vi "Affichage - 2 cam - 1P - 2.vi"(7 "Image 2D 2":picture, 8 "Couleur rectangle":u32(colorbox)=16775680, 9 "Caméra D":T1, 10 "Choix cam":u16, 11 "Caméra G":T1) -> (2 "Image 2D":picture)   [LabVIEW 2013]
panel:
  # "Affichage"
  # "Pour un rectangle"
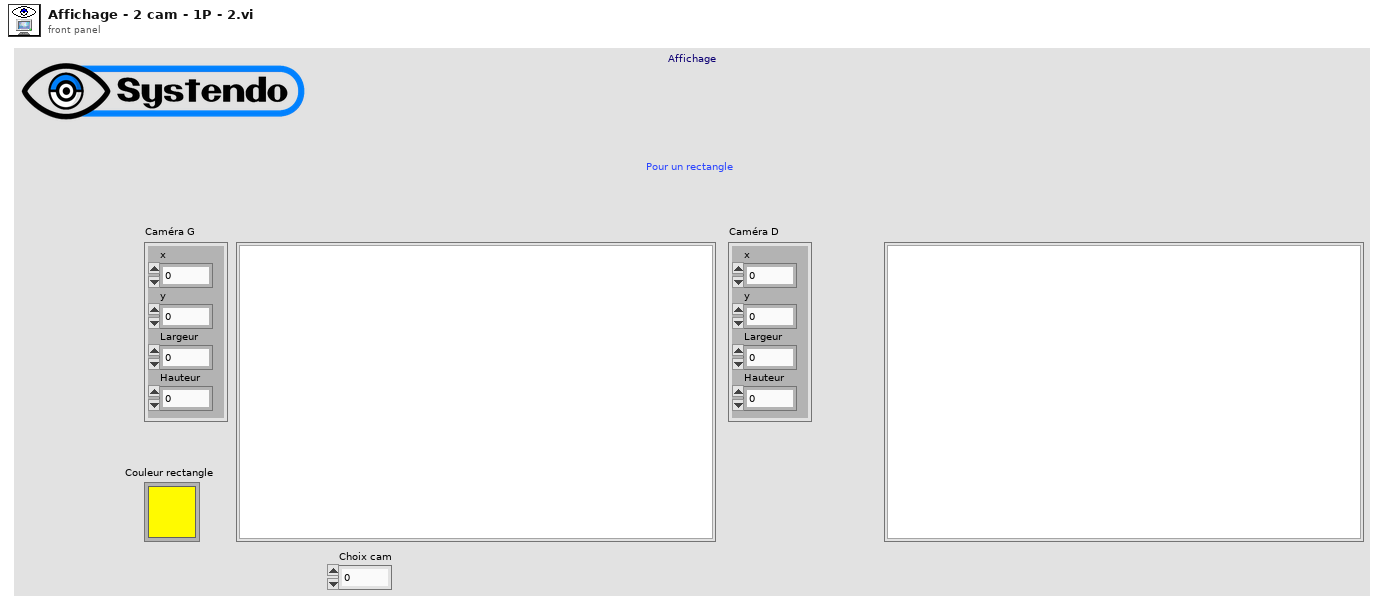
[diagram p1: front panel]
types:
  T1 = cluster{"x":i16, "y":i16, "Largeur":i16, "Hauteur":i16}
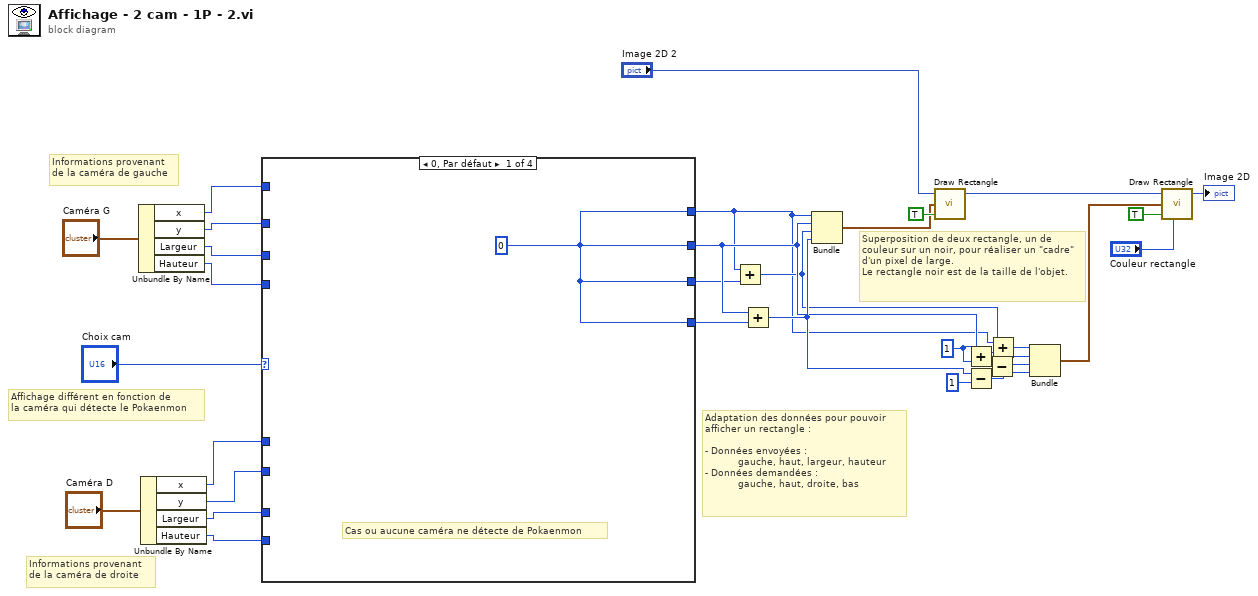
[diagram p0: block diagram]
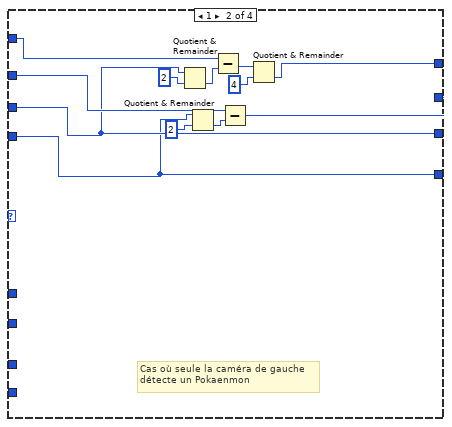
[diagram p2: hidden frame]
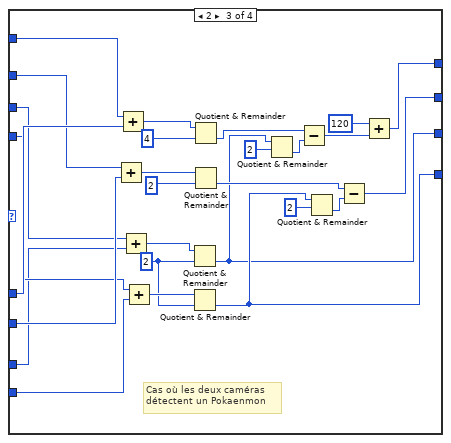
[diagram p3: hidden frame]
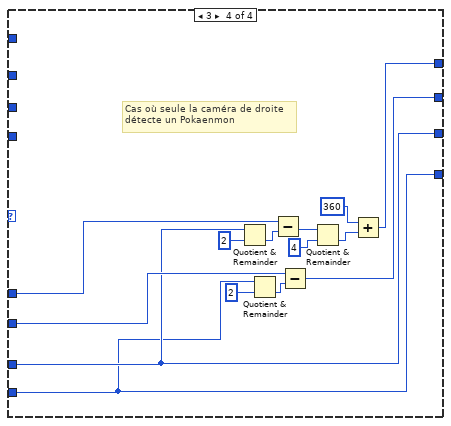
[diagram p4: hidden frame]
diagram:
  w10 = i16 1 ("y")
  w7 = i16 1 ("y")
  # "Superposition de deux rectangle, un de couleur sur un noir, pour réaliser un \"cadre\" d'un pixel de large.\nLe rectangle noir est de la taille de l'objet."
  # "Adaptation des données pour pouvoir\nafficher un rectangle :\n\n- Données envoyées :\n           gauche, haut, largeur, hauteur\n- Données demandées :\n           gauche, haut, droite, bas"
  # "Informations provenant\nde la caméra de droite"
  # "Informations provenant\nde la caméra de gauche"
  # "Affichage différent en fonction de\nla caméra qui détecte le Pokaenmon"
  n1 = Unbundle By Name("Caméra G") -> ("x"=w23:i16, "y"=w22:i16, "Largeur"=w21:i16, "Hauteur"=w20:i16)
  n2 = Unbundle By Name("Caméra D") -> ("x"=w16:i16, "y"=w17:i16, "Largeur"=w18:i16, "Hauteur"=w19:i16)
  n3 = case shown="0, Par défaut" "Choix cam" {
    tunnel: [w32 w36 w54 w81] -> w27
    tunnel: [w32 w42 w53 w83] -> w30
    tunnel: [w32 w40 w45 w76] -> w26
    tunnel: [w32 w34 w51 w73] -> w29
    tunnel: w16 -> [_ _ w64 w84]
    tunnel: w17 -> [_ _ w62 w85]
    tunnel: w18 -> [_ _ w59 w76]
    tunnel: w19 -> [_ _ w61 w73]
    tunnel: w20 -> [_ w34 w60 _]
    tunnel: w21 -> [_ w40 w58 _]
    tunnel: w22 -> [_ w43 w63 _]
    tunnel: w23 -> [_ w44 w65 _]
    frame 0, Default {
      w32 = 0
      # "Cas ou aucune caméra ne détecte de Pokaenmon"
    }
    frame 1 {
      # "Cas où seule la caméra de gauche\ndétecte un Pokaenmon"
      n4 = Quotient & Remainder(x=w40, y=u16 2) -> (floor(x/y)=w39:u16)  [unwired: 1 out]
      n5 = Quotient & Remainder(x=w34, y=u16 2) -> (floor(x/y)=w33:u16)  [unwired: 1 out]
      n6 = Subtract(x=w44, y=w39) -> (x-y=w37:u16)
      n7 = Subtract(x=w43, y=w33) -> (x-y=w42:u16)
      n8 = Quotient & Remainder(x=w37, y=u16 4) -> (floor(x/y)=w36:u16)  [unwired: 1 out]
    }
    frame 2 {
      w66 = i16 2 ("y")
      # "Cas où les deux caméras\ndétectent un Pokaenmon"
      n9 = Add(x=w63, y=w62) -> (x+y=w70:i16)
      n10 = Add(x=w65, y=w64) -> (x+y=w71:i16)
      n11 = Add(x=w58, y=w59) -> (x+y=w68:i16)
      n12 = Add(x=w60, y=w61) -> (x+y=w67:i16)
      n13 = Quotient & Remainder(x=w68, y=w66) -> (floor(x/y)=w45:i16)  [unwired: 1 out]
      n14 = Quotient & Remainder(x=w67, y=w66) -> (floor(x/y)=w51:i16)  [unwired: 1 out]
      n15 = Quotient & Remainder(x=w71, y=i16 4) -> (floor(x/y)=w47:i16)  [unwired: 1 out]
      n16 = Quotient & Remainder(x=w70, y=i16 2) -> (floor(x/y)=w56:i16)  [unwired: 1 out]
      n17 = Quotient & Remainder(x=w45, y=u16 2) -> (floor(x/y)=w48:u16)  [unwired: 1 out]
      n18 = Subtract(x=w47, y=w48) -> (x-y=w46:u16)
      n19 = Quotient & Remainder(x=w51, y=u16 2) -> (floor(x/y)=w50:u16)  [unwired: 1 out]
      n20 = Subtract(x=w56, y=w50) -> (x-y=w53:u16)
      n21 = Add(x=u16 120, y=w46) -> (x+y=w54:u16)
    }
    frame 3 {
      # "Cas où seule la caméra de droite\ndétecte un Pokaenmon"
      n22 = Quotient & Remainder(x=w76, y=u16 2) -> (floor(x/y)=w75:u16)  [unwired: 1 out]
      n23 = Quotient & Remainder(x=w73, y=u16 2) -> (floor(x/y)=w72:u16)  [unwired: 1 out]
      n24 = Subtract(x=w84, y=w75) -> (x-y=w79:u16)
      n25 = Subtract(x=w85, y=w72) -> (x-y=w83:u16)
      n26 = Quotient & Remainder(x=w79, y=u16 4) -> (floor(x/y)=w78:u16)  [unwired: 1 out]
      n27 = Add(x=u16 360, y=w78) -> (x+y=w81:u16)
    }
  }
  n28 = Add(x=w27, y=w26) -> (x+y=w28:i32)
  n29 = Add(x=w30, y=w29) -> (x+y=w31:i32)
  n30 = Bundle(w27, w30, w28, w31) -> (w2:cluster{i32, i32, i32, i32})  [unwired: 1 in]
  n31 = call <vilib>:"Draw Rectangle.vi"("picture"="Image 2D 2", "rect"=w2, "fill?(F)"=TRUE) -> ("new picture"=w13:picture)  [unwired: 6 in]
  n32 = Add(x=w30, y=w7) -> (x+y=w6:i32)
  n33 = Subtract(x=w31, y=w10) -> (x-y=w9:i32)
  n34 = Subtract(x=w28, y=w10) -> (x-y=w8:i32)
  n35 = Add(x=w27, y=w7) -> (x+y=w5:i32)
  n36 = Bundle(w5, w6, w8, w9) -> (w11:cluster{i32, i32, i32, i32})  [unwired: 1 in]
  n37 = call <vilib>:"Draw Rectangle.vi"("picture"=w13, "rect"=w11, "fill?(F)"=TRUE, "color(black)"="Couleur rectangle") -> ("new picture"=→"Image 2D":picture)  [unwired: 5 in]
